vi "GetCellStrColor.vi"(7 "Color":u32, 8 "error in (no error)":errorcluster, 10 "Hdr Name":T1, 11 "Resistance in":refnum<class "Resistance.lvclass">) -> (0 "error out":errorcluster, 1 "Cell String":string, 2 "Cell Color":u32, 3 "Resistance out":refnum<class "Resistance.lvclass">)   [LabVIEW 2018, in "Measurement Channels.lvlib" / "Resistance.lvclass"]
uses:
  Resistance.lvclass
  Common/Controls/HeaderNames.ctl
  SubVIs Table/Custom Ctls Table/ge_ColType.ctl
  Resistance.lvclass/Resistance.ctl
  Class Channel/Channel.lvclass
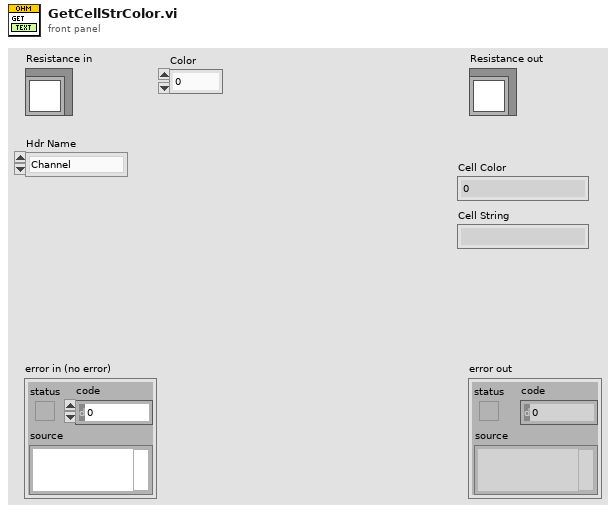
[diagram p1: front panel]
types:
  T1 = typedef "HeaderNames.ctl" = enum16{"Channel", "Device", "Spacer", "Description", "MB", "Range", "Terminal", "Coupling", "Thresh (V)", "Pulse/Rev", "Slope", "Min EU", "Min RPM", "mV/EU", "Iex", "Temp Units", "Type", "CJC Src", "CJC Val", "Ro", "Wire Cfg", "Strain Mode", "Vex", "Bridge Type", "GF", "Gauge Res", "Poisson", "Lead Res", "Init Strain", "GAF", "Scale", "Offset", "Unit (EU)", "dB?", "dB Ref", "Cal Mag", "Cal Units", "Max Temp", "Min Temp", "Max Strain", "Min Strain"}
  T2 = typedef "ge_ColType.ctl" = enum16{"Volts", "Amps", "Ohms", "TermCfg", "WireCfg", "Coup", "Slope", "Iex", "CalUnits", "ThrmUnits", "ThrmType", "CJCSrc", "BrdgType", "Strn Mode", "RTDType"}
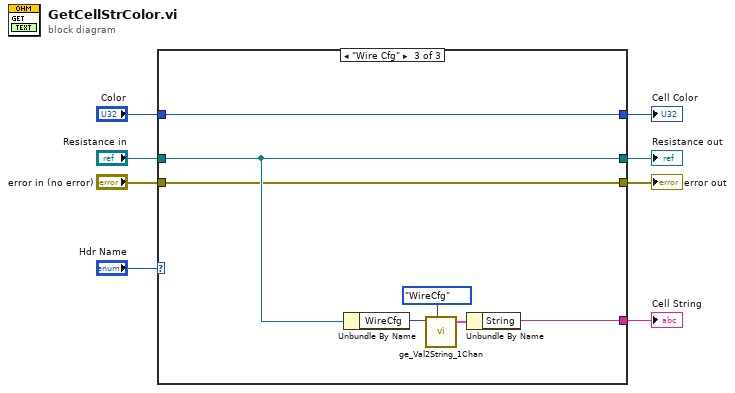
[diagram p0: block diagram]
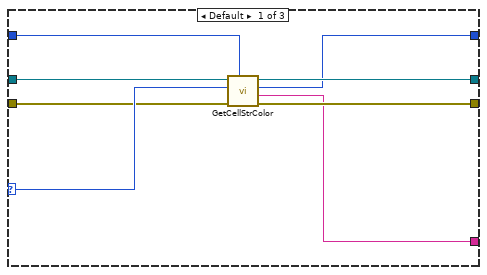
[diagram p2: hidden frame]
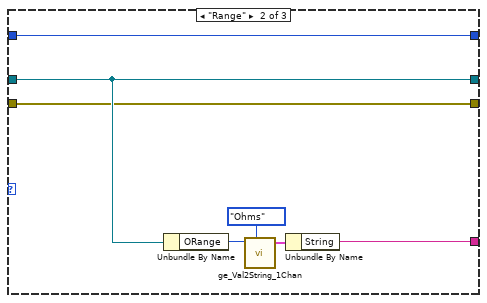
[diagram p3: hidden frame]
diagram:
  n1 = case shown="\"Wire Cfg\"" "Hdr Name" {
    selector: "Hdr Name" -> [w12 _ _]
    tunnel: "Resistance in" -> [w16 w18 w25]
    tunnel: [w9 w21 w28] -> w2
    tunnel: [w14 w19 w26] -> w5
    tunnel: "Color" -> [w13 w19 w26]
    tunnel: [w15 w18 w25] -> w7
    tunnel: "error in (no error)" -> [w11 w17 w24]
    tunnel: [w10 w17 w24] -> w3
    frame Default {
      n2 = call-parent "GetCellStrColor.vi"("Color"=w13, "error in (no error)"=w11, "Hdr Name"=w12, "Channel in"=w16) -> ("error out"=w10:errorcluster, "Cell String"=w9:string, "Cell Color"=w14:u32, "Channel out"=w15:refnum<class "Resistance.lvclass">)  [unwired: 4 in]
    }
    frame "Range" {
      n3 = Unbundle By Name(w18) -> ("ORange"=w20:u16)
      n4 = call "ge_Val2String_1Chan.vi"("Value"=w20, "ColType"=ge_ColType."Ohms") -> ("String and Val"=w22:cluster{"String":string, "Value":u16})  [unwired: 5 in]
      n5 = Unbundle By Name(w22) -> ("String"=w21:string)
    }
    frame "Wire Cfg" {
      n6 = Unbundle By Name(w25) -> ("WireCfg"=w27:u16)
      n7 = call "ge_Val2String_1Chan.vi"("Value"=w27, "ColType"=ge_ColType."WireCfg") -> ("String and Val"=w29:cluster{"String":string, "Value":u16})  [unwired: 5 in]
      n8 = Unbundle By Name(w29) -> ("String"=w28:string)
    }
  }
  "error out" <- w3
  "Resistance out" <- w7
  "Cell String" <- w2
  "Cell Color" <- w5
